vi "Log.vi"(8 "error in (no error)":errorcluster, 11 "SCADA in":refnum<class "SCADA.lvclass">) -> (0 "error out":errorcluster, 3 "SCADA out":refnum<class "SCADA.lvclass">)   [LabVIEW 2015, in "SCADA Core.lvlib" / "SCADA.lvclass"]
uses:
  SCADA.lvclass
  SCADA.lvclass/SCADA.ctl
  Logger Actor/Logger Messages/Log Measurements Msg/Log Measurements Msg.lvclass/Log Measurements Msg.ctl
  <vilib>/ActorFramework/Message Enqueuer/Message Enqueuer.lvclass/Message Enqueuer.ctl
  Logger Actor/Logger Messages/Log Setpoints Msg/Log Setpoints Msg.lvclass/Log Setpoints Msg.ctl
  <vilib>/ActorFramework/Message Enqueuer/Enqueue.vi
  <vilib>/ActorFramework/Message Priority Queue/Priority Enqueue.vi
  Logger Actor/Logger Messages/Log Measurements Msg/Log Measurements Msg.lvclass
  Logger Actor/Logger Messages/Log Setpoints Msg/Log Setpoints Msg.lvclass
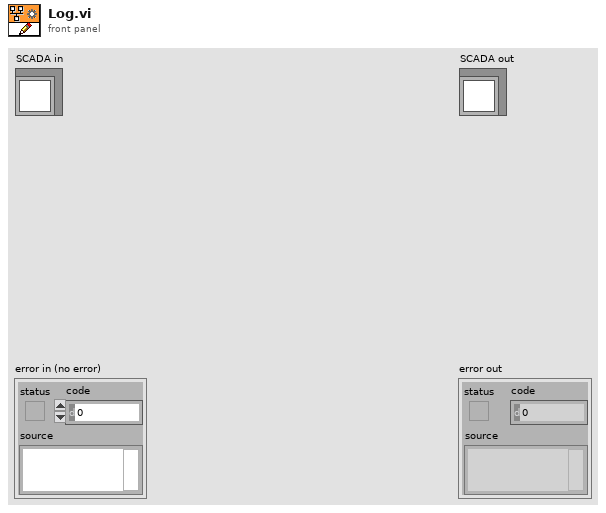
[diagram p1: front panel]
types:
  T1 = typedef "Tools_KeyedArray.lvlib/KeyedArray.ctl" = cluster{"keys":string[], "values":string[]}
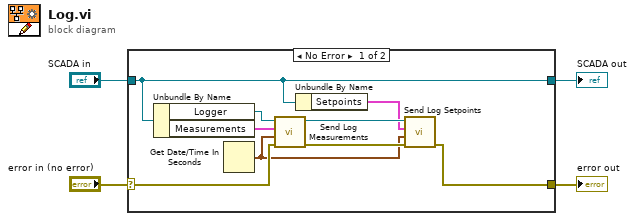
[diagram p0: block diagram]
diagram:
  n1 = case shown="No Error" "error in (no error)" {
    selector: "error in (no error)" -> [w11 w15]
    tunnel: [w5 w15] -> w3
    tunnel: [w8 w14] -> w1
    tunnel: "SCADA in" -> [w8 w14]
    frame No Error {
      n2 = Unbundle By Name(w8) -> ("Logger"=w13:refnum<class "Message Enqueuer.lvclass">, "Measurements"=w12:T1)
      n3 = Get Date/Time In Seconds() -> (seconds since 1Jan1904=w6:timestamp)
      n4 = call "Send Log Measurements.vi"("error in (no error)"=w11, "Time Stamp"=w6, "Measurements"=w12, "Message Enqueuer"=w13) -> ("error out"=w9:errorcluster, "Message Enqueuer out"=w10:refnum<class "Message Enqueuer.lvclass">)  [unwired: 6 in]
      n5 = Unbundle By Name(w8) -> ("Setpoints"=w7:T1)
      n6 = call "Send Log Setpoints.vi"("error in (no error)"=w9, "Time Stamp"=w6, "Setpoints"=w7, "Message Enqueuer"=w10) -> ("error out"=w5:errorcluster)  [unwired: 6 in, 1 out]
    }
    frame Error {
    }
  }
  "error out" <- w3
  "SCADA out" <- w1
